vi "Generate rel times path.vi"(11 "Binary file to read":path) -> (1 "Relative times file not found or error":bool, 2 "Relative times file path":path)   [LabVIEW 2020]
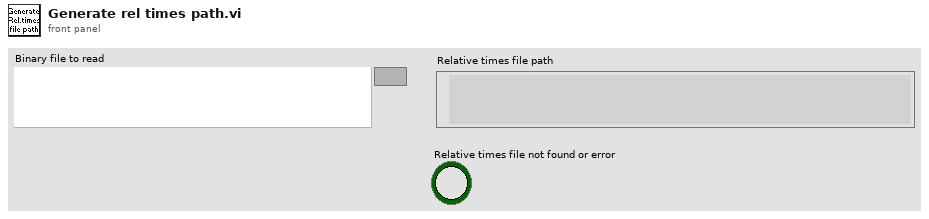
[diagram p1: front panel]
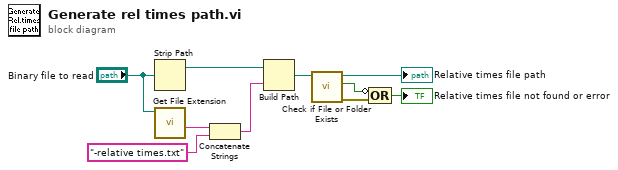
[diagram p0: block diagram]
diagram:
  n1 = Strip Path(path="Binary file to read") -> (stripped path=w7:path)  [unwired: 1 out]
  n2 = call <vilib>:"Get File Extension.vi"("file"="Binary file to read") -> ("filename without extension"=w9:string)  [unwired: 6 in, 4 out]
  n3 = Concatenate Strings(w9, "-relative times.txt" ("string")) -> (w6:string)
  n4 = Build Path(base path=w7, name or relative path=w6) -> (appended path=w5:path)
  n5 = call <vilib>:"Check if File or Folder Exists.vi"("path"=w5) -> ("error out"=w2:errorcluster, "file or folder exists?"=w3:bool, "dup path"=→"Relative times file path":path)  [unwired: 8 in]
  n6 = Compound Arithmetic op=OR(invert w3, w2) -> (→"Relative times file not found or error":bool)
